vi "VD-Connect.vi"(8 "error in (no error)":errorcluster, 11 "VD-LV-LiteVNA in":refnum<class "VD-LV-LiteVNA.lvclass">) -> (0 "error out":errorcluster, 3 "VD-LV-LiteVNA out":refnum<class "VD-LV-LiteVNA.lvclass">)   [LabVIEW 2020, in "VD-LV-LiteVNA.lvclass"]
uses:
  VD-LV-LiteVNA.lvclass
  hardware-protocol/serial/HP-S-settings.ctl
  hardware-protocol/serial/HP-S-baudrate.ctl
  VD-action.ctl
  VD-LV-LiteVNA.lvclass/VD-LV-LiteVNA.ctl
  hardware-protocol/serial/HP-S-Serial.lvclass
panel:
  out "x = y?":bool
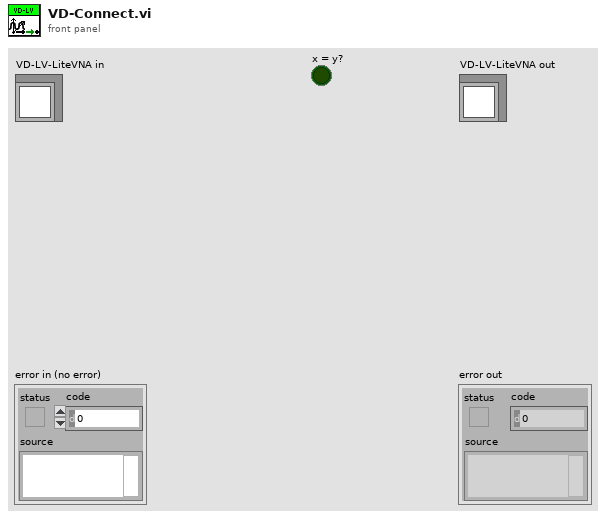
[diagram p1: front panel]
types:
  T1 = typedef "VD-LV-LiteVNA.lvclass/VD-action.ctl" = enum16{"checkCom", "SweepStartHz", "SweepStopHz", "SweepPoints", "valuesPerFrequency", "RawSamplesMode", "ValuesFIFO", "deviceVariant", "protocolVersion", "hardwareRevision", "firmwareMajor", "firmwareMinor"}
  T2 = typedef "HP-S-Serial.lvclass/HP-S-settings.ctl" = cluster{"VISA resource name":refnum<visa-resource-name>, "baud rate (9600)":T3, "timeout (10sec)":u32, "termination char\n(0xA = '\\n' = LF) ":u8, "Enable Termination\nChar (T)":bool, "data bits (8)":u16, "parity (0:none)":enum16{"None", "Odd", "Even", "Mark", "Space"}}
  T3 = typedef "HP-S-Serial.lvclass/HP-S-baudrate.ctl" = u32
  T4 = typedef "HP-S-Serial.lvclass/HP-S-data.ctl" = u8[]
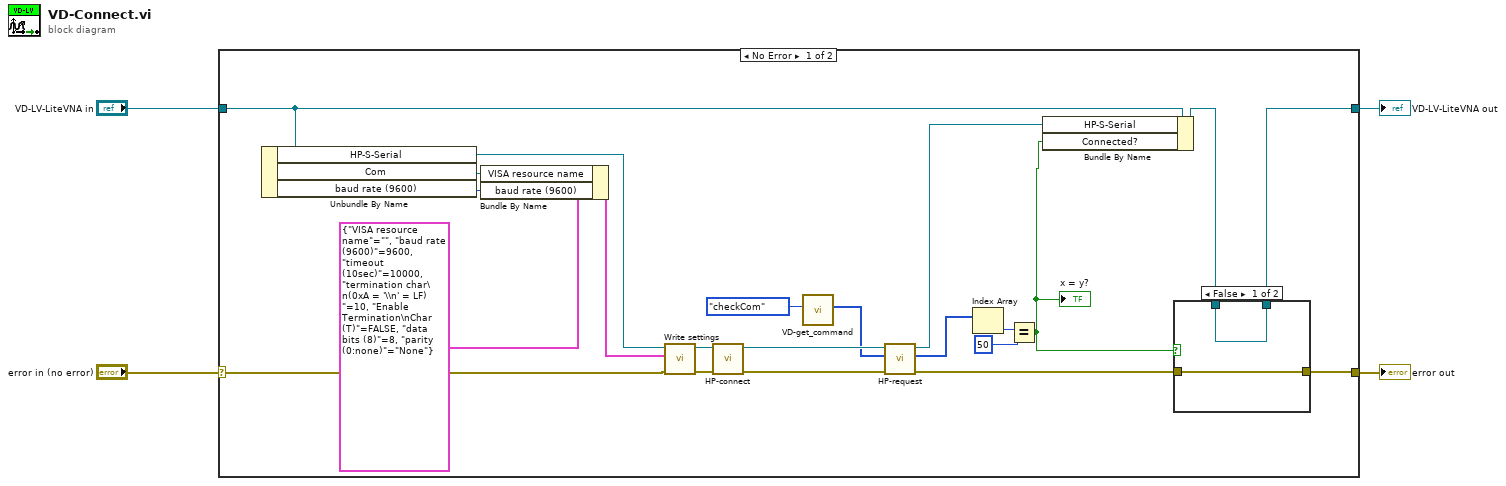
[diagram p0: block diagram]
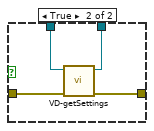
[diagram p2: hidden frame]
diagram:
  n1 = case shown="No Error" "error in (no error)" {
    selector: "error in (no error)" -> [w20 w34]
    tunnel: [w8 w34] -> w3
    tunnel: [w6 w33] -> w1
    tunnel: "VD-LV-LiteVNA in" -> [w26 w33]
    frame No Error {
      n2 = Unbundle By Name(w26) -> ("HP-S-Serial"=w25:refnum<class "HP-S-Serial.lvclass">, "Com"=w22:refnum<visa-resource-name>, "baud rate (9600)"=w21:T3)
      n3 = Bundle By Name(cluster=T2 {"VISA resource name"="", "baud rate (9600)"=9600, "timeout (10sec)"=10000, "termination char\n(0xA = '\\n' = LF) "=10, "Enable Termination\nChar (T)"=FALSE, "data bits (8)"=8, "parity (0:none)"=enum."None"} ("settings"), "VISA resource name"=w22, "baud rate (9600)"=w21) -> (w23:T2)
      n4 = call-dynamic "Write settings.vi"("error in (no error)"=w20, "settings"=w23, "HP-S-Serial in"=w25) -> ("error out"=w18:errorcluster, "HP-S-Serial out"=w19:refnum<class "HP-S-Serial.lvclass">)  [unwired: 7 in]
      n5 = call-dynamic "HP-connect.vi"("error in (no error)"=w18, "HP-S-Serial in"=w19) -> ("error out"=w16:errorcluster, "HP-S-Serial out"=w17:refnum<class "HP-S-Serial.lvclass">)  [unwired: 8 in]
      n6 = call "VD-get_command.vi"("action"=VD-action."checkCom") -> ("Command"=w13:T4)  [unwired: 10 in]
      n7 = call-dynamic "HP-request.vi"("error in (no error)"=w16, "write buffer"=w13, "HP-S-Serial in"=w17) -> ("error out"=w9:errorcluster, "read buffer"=w12:T4, "HP-S-Serial out"=w15:refnum<class "HP-S-Serial.lvclass">)  [unwired: 6 in]
      n8 = Index Array(array=w12) -> (element=w11:u8)  [unwired: 1 in]
      n9 = Equal?(x=w11, y=u8 50) -> (x = y?=w5:bool)
      "x = y?" <- w5
      n10 = Bundle By Name(cluster=w26, "HP-S-Serial"=w15, "Connected?"=w5) -> (w7:refnum<class "VD-LV-LiteVNA.lvclass">)
      n11 = case shown="False" w5 {
        tunnel: w9 -> [w28 w32]
        tunnel: [w28 w31] -> w8
        tunnel: w7 -> [w27 w30]
        tunnel: [w27 w29] -> w6
        frame False {
        }
        frame True {
          n12 = call "VD-getSettings.vi"("error in (no error)"=w32, "VD-LV-LiteVNA in"=w30) -> ("error out"=w31:errorcluster, "VD-LV-LiteVNA out"=w29:refnum<class "VD-LV-LiteVNA.lvclass">)  [unwired: 7 in, 1 out]
        }
      }
    }
    frame Error {
    }
  }
  "error out" <- w3
  "VD-LV-LiteVNA out" <- w1
